vi "Forward Kinematics.vi"(8 "error in (no error)":errorcluster, 10 "joint positions":dbl[](array[numeric]), 11 "Robot Arm in":refnum<class "Robot Arm.lvclass">) -> (0 "error out":errorcluster, 2 "end effector transform":T1, 3 "Robot Arm out":refnum<class "Robot Arm.lvclass">)   [LabVIEW 2013, in "Kinematics.lvlib"]
uses:
  Kinematics.lvlib
  <vilib>/Analysis/Matrix/Datatypes/RealMatrix.ctl
  Robot Arm.lvclass
  Robot Arm.lvclass/Robot Arm.ctl
  Link/Link.lvclass/Link.ctl
  <vilib>/Analysis/baseanly.llb/Real A x B.vi
  <vilib>/Analysis/Matrix/Numeric/Conversions/Array To Matrix.vi
  <vilib>/Analysis/Matrix/Numeric/Conversions/Array To Matrix - RA.vi
  Link/Skew.vi
  <vilib>/Analysis/Matrix/Numeric/Conversions/Array To Matrix - RA2.vi
  <vilib>/Analysis/Matrix/Numeric/Multiply/Multiply.vi
  <vilib>/Analysis/Matrix/Numeric/Multiply/Multiply - R,RM.vi
  <vilib>/Analysis/Matrix/Numeric/Multiply/Multiply - RM,RM.vi
  <vilib>/Analysis/Matrix/Numeric/Multiply/Multiply - RM,R.vi
  <vilib>/Analysis/Matrix/Numeric/Add/Add.vi
  <vilib>/Analysis/Matrix/Numeric/Add/Add - RM,RM.vi
  <vilib>/Analysis/Matrix/Numeric/Subtract/Subtract.vi
  <vilib>/Analysis/Matrix/Numeric/Subtract/Subtract - RM,RM.vi
  Link/Link.lvclass
  <vilib>/robotics/Utilities/NI_Robotics Utilities.lvlib
  <vilib>/Analysis/NI_AALBase.lvlib
  <vilib>/Analysis/Matrix/NI_Matrix.lvlib
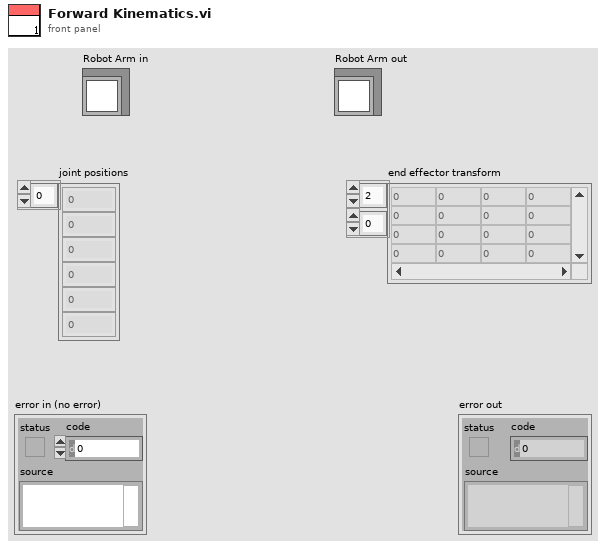
[diagram p1: front panel]
types:
  T1 = typedef "NI_Matrix.lvlib/RealMatrix.ctl" = dbl[][]
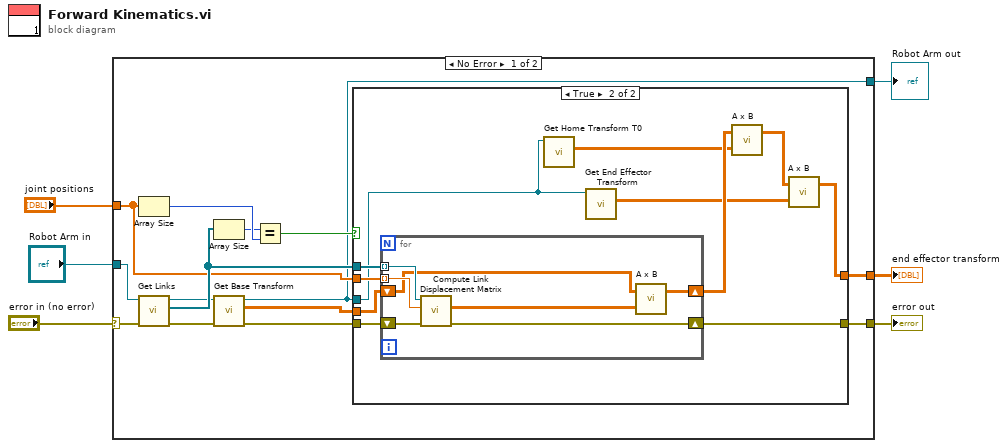
[diagram p0: block diagram]
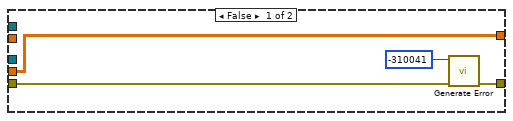
[diagram p2: hidden frame]
diagram:
  n1 = case shown="No Error" "error in (no error)" {
    selector: "error in (no error)" -> [w13 w44]
    tunnel: [w20 w44] -> w5
    tunnel: [w10 w43] -> w2
    tunnel: "joint positions" -> [w17 _]
    tunnel: [w19 _] -> w3
    tunnel: "Robot Arm in" -> [w12 w43]
    frame No Error {
      n2 = Array Size(array=w17) -> (size(s)=w16:i32)
      n3 = call "Get Links.vi"("error in (no error)"=w13, "Robot Arm in"=w12) -> ("error out"=w8:errorcluster, "Links"=w18:refnum<class "Link.lvclass">[], "Robot Arm out"=w9:refnum<class "Robot Arm.lvclass">)  [unwired: 7 in]
      n4 = Array Size(array=w18) -> (size(s)=w15:i32)
      n5 = call "Get Base Transform.vi"("error in (no error)"=w8, "Robot Arm in"=w9) -> ("error out"=w11:errorcluster, "Base Transform"=w7:T1, "Robot Arm out"=w10:refnum<class "Robot Arm.lvclass">)  [unwired: 7 in]
      n6 = Equal?(x=w15, y=w16) -> (x = y?=w14:bool)
      n7 = case shown="True" w14 {
        tunnel: [w22 w35] -> w20
        tunnel: [w24 w30] -> w19
        tunnel: w11 -> [w23 w26]
        tunnel: w7 -> [w24 w25]
        tunnel: w18 -> [_ w33]
        tunnel: w17 -> [_ w32]
        tunnel: w10 -> [_ w29]
        frame False {
          n8 = call <vilib>:"Generate Error.vi"("error in (no error)"=w23, "code"=-310041) -> ("error out"=w22:errorcluster)  [unwired: 9 in]
        }
        frame True {
          n9 = for {
            tunnel: w33 -> [w42] mode=indexing
            shift-right: [w36] -> w34
            shift-left: w25 -> [w38]
            tunnel: w32 -> [w41] mode=indexing
            shift-right: [w40] -> w35
            shift-left: w26 -> [w39]
            n10 = call "Compute Link Displacement Matrix.vi"("error in (no error)"=w39, "q"=w41, "Link in"=w42) -> ("error out"=w40:errorcluster, "Displacement Matrix"=w37:T1)  [unwired: 6 in, 1 out]
            n11 = call-poly <vilib>:"A x B.vi"("B"=w37, "A"=w38) -> ("A x B"=w36:T1)  [unwired: 1 out]
          }
          n12 = call "Get Home Transform T0.vi"("Robot Arm in"=w29) -> ("T0 Transform"=w28:T1)  [unwired: 8 in, 2 out]
          n13 = call "Get End Effector Transform.vi"("Robot Arm in"=w29) -> ("End Effector Transform"=w27:T1)  [unwired: 8 in, 2 out]
          n14 = call-poly <vilib>:"A x B.vi"("B"=w28, "A"=w34) -> ("A x B"=w31:T1)  [unwired: 1 out]
          n15 = call-poly <vilib>:"A x B.vi"("B"=w27, "A"=w31) -> ("A x B"=w30:T1)  [unwired: 1 out]
        }
      }
    }
    frame Error {
    }
  }
  "error out" <- w5
  "end effector transform" <- w3
  "Robot Arm out" <- w2
